vi "SubsystemStör.vi"() -> (2 "Fsx":dbl)   [LabVIEW 2013]
uses:
  <vilib>/Simulation/Implementation/Shared/SIMSCR Execution Mode.ctl
  <vilib>/Simulation/Scripting/Companion Diagram/SimConfigNode/SimParams.ctl
  <vilib>/Simulation/Scripting/Companion Diagram/SimConfigNode/_simSolvers.ctl
  <vilib>/Simulation/Param Hierarchy/Typedefs/SIMPH Param Control Actions.ctl
  <vilib>/Simulation/Implementation/Shared/NILVSim_ParamChanged.vi
  <vilib>/Simulation/Implementation/Shared/NILVSIM_BeginStep.vi
  <vilib>/Simulation/SignalArithmetic/Implementation/NILVSim Gain.llb/SIM Gain (scalar).vi
  <vilib>/Simulation/Implementation/Shared/NILVSim_Manager.vi
  <vilib>/Simulation/Implementation/Shared/NILVSim_FinalizeModel.vi
  <vilib>/Simulation/Implementation/Shared/SIM Unbundle Sim Info.vi
  <vilib>/Utility/error.llb/Clear Errors.vi
  <vilib>/Simulation/Implementation/Shared/NILVSim_GetModelError.vi
  <vilib>/Simulation/Implementation/Shared/SIM SimErrorHandler.vi
  <vilib>/Simulation/Implementation/Shared/SIM Bundle Sim Info.vi
  geschwindigkeit.vi
  p''.vi
  p.vi
  p'.vi
  <vilib>/Simulation/Implementation/Shared/NILVSim_Initialize.vi
  <vilib>/Simulation/Utility/Implementation/NILVSim Get Time and IsAcceptedStep.vi
  <vilib>/Simulation/Implementation/Shared/SIMSH Read Queue.vi
  <vilib>/Simulation/Scripting/Companion Diagram/SimConfigNode/SimDog.xnode
  <vilib>/Simulation/Implementation/XNodeFramework/SimXNode/SimX.xnode
  <vilib>/Simulation/Implementation/Shared/NI_SIM_Implementation.lvlib
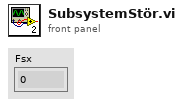
[diagram p1: front panel]
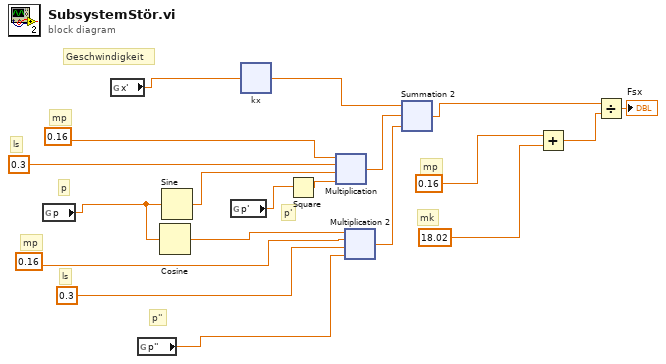
[diagram p0: block diagram]
diagram:
  # "mp"
  # "ls"
  # "mp"
  # "Geschwindigkeit"
  # "p'"
  # "p''"
  # "p"
  # "mk"
  # "ls"
  # "mp"
  n1 = global read "p.vi" "p"() -> (w17:dbl)
  n2 = global read "geschwindigkeit.vi" "x'"() -> (w19:dbl)
  n3 = global read "p''.vi" "p''"() -> (w18:dbl)
  n4 = Cosine ("Cosinus")(x=w17) -> (cos(x)=w6:dbl)
  n5 = Sine ("Sinus")(x=w17) -> (sin(x)=w2:dbl)
  n6 = global read "p'.vi" "p'"() -> (w16:dbl)
  n7 = xnode "kx"("input"=w19) -> ("output"=w15:dbl)  [unwired: 3 in]
  n8 = Square ("Quadrat")(x=w16) -> (x^2=w3:dbl)
  n9 = xnode ("Multiplication")("Operand1"=0.16 ("Constant"), "Operand2"=0.3 ("Constant 3"), "Operand3"=w2, "Operand4"=w3) -> ("Result"=w4:dbl)
  n10 = xnode ("Multiplication 2")("Operand1"=w6, "Operand2"=0.16 ("Constant 6"), "Operand3"=0.3 ("Constant 5"), "Operand4"=w18) -> ("Result"=w5:dbl)
  n11 = xnode ("Summation 2")("Operand1"=w15, "Operand2"=w4, "Operand3"=w5) -> ("Result"=w7:dbl)
  n12 = Add ("Addieren 2")(x=0.16 ("Constant 4"), y=18.02 ("Constant 2")) -> (x+y=w8:dbl)
  n13 = Divide(x=w7, y=w8) -> (x/y=→"Fsx":dbl)
